vi "RT Main.vi"() -> ()   [LabVIEW 2021]
doc: "This example monitors the myRIO onboard button and increments or decrements the number below based on the Direction control."
uses:
  <vilib>/myRIO/Instrument Drivers/Utilities/Utilities.lvlib
  <vilib>/myRIO/Express VI/Onboard Devices/Button/Button Express VI.xnode
  <vilib>/myRIO/Instrument Drivers/Onboard IO/DIO/vis/Read.vi
  <vilib>/myRIO/Instrument Drivers/Onboard IO/DIO/DIO.lvlib
  <vilib>/myRIO/Common/Instrument Driver Framework/myRIO v1.0/DIO/typedefs/DIO Channels Enum.ctl
  <vilib>/myRIO/Common/Instrument Driver Framework/myRIO v1.0/DIO/typedefs/DIO Channels List.ctl
  <vilib>/myRIO/Common/Instrument Driver Framework/Utilities/typedefs/Generic FPGA Reference.ctl
  <vilib>/myRIO/Common/Instrument Driver Framework/Utilities/typedefs/myRIO v1.0 Reference.ctl
  <vilib>/myRIO/Common/Instrument Driver Framework/Utilities/typedefs/Hardware Version Enum.ctl
  <vilib>/myRIO/Common/Instrument Driver Framework/Utilities/typedefs/myRIO Generic Hardware Reference.ctl
  <vilib>/myRIO/Instrument Drivers/Onboard IO/DIO/typedefs/DIO Reference.ctl
  <vilib>/myRIO/Instrument Drivers/Onboard IO/DIO/vis/myRIO DIO Open.xnode
  <vilib>/myRIO/Common/Instrument Driver Framework/Utilities/vis/Is FPGA Ref Available.vi
  <vilib>/myRIO/Common/Instrument Driver Framework/myRIO v1.0/DIO/vis/myRIO v1.1 Open DIO.vi
  <vilib>/userdefined/High Color/nirio_resource_hc.ctl
panel:
  out "error out":errorcluster
  out "Button Value":bool
  in  "Direction":bool
  in  "Stop":bool
  out "Up/Down Counter":i32
  # "Overview: This example monitors the myRIO onboard button and increments or decrements the number below based on the Direction control.\nInstructions:\n1. Check the myRIO target IP Address in the project and make sure the target IP Address is correct.\n2. Run the VI.\n3. Push the button on the myRIO device."
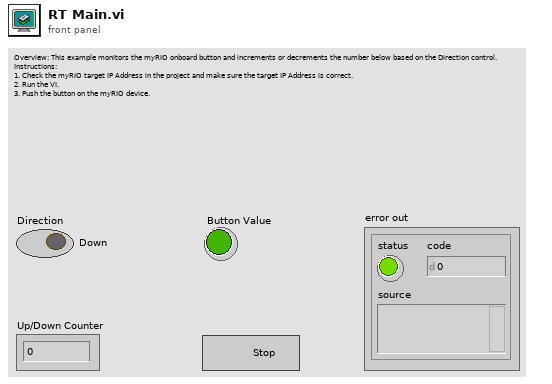
[diagram p1: front panel]
types:
  T1 = typedef "DIO.lvlib/DIO Reference.ctl" = cluster{"myRIO Reference":T2, "DIO Channels List":T6}
  T2 = typedef "myRIO Generic Hardware Reference.ctl" = cluster{"myRIO Model":T3, "myRIO Hardware Reference":T4}
  T3 = typedef "Hardware Version Enum.ctl" = enum16{"Unknown", "myRIO-1900", "myRIO-1950", "roboRIO", "NI ELVIS RIO CM", "ELVIS III"}
  T4 = typedef "myRIO v1.0 Reference.ctl" = cluster{"Generic FPGA Reference":T5, "Allow multiple opens":bool}
  T5 = typedef "Generic FPGA Reference.ctl" = refnum<k20>
  T6 = typedef "DIO Channels List.ctl" = T7[]
  T7 = typedef "DIO Channels Enum.ctl" = enum16{"Not Connected", "C/DIO0", "C/DIO1", "C/DIO2", "C/DIO3", "C/DIO4", "C/DIO5", "C/DIO6", "C/DIO7", "A/DIO0", "A/DIO1", "A/DIO2", "A/DIO3", "A/DIO4", "A/DIO5", "A/DIO6", "A/DIO7", "A/DIO8", "A/DIO9", "A/DIO10", "A/DIO11", "A/DIO12", "A/DIO13", "A/DIO14", "A/DIO15", "A/DIO16", "A/DIO17", "A/DIO18", "A/DIO19", "B/DIO0", "B/DIO1", "B/DIO2", "B/DIO3", "B/DIO4", "B/DIO5", "B/DIO6", "B/DIO7", "B/DIO8", "B/DIO9", "B/DIO10", "B/DIO11", "B/DIO12", "B/DIO13", "B/DIO14", "B/DIO15", "B/DIO16", "B/DIO17", "B/DIO18", "B/DIO19", "LED0", "LED1", "LED2", "LED3", "Button0", "DIO/DIO0", "DIO/DIO1", "DIO/DIO2", "DIO/DIO3", "DIO/DIO4", "DIO/DIO5", "DIO/DIO6", "DIO/DIO7", "DIO/DIO8", "DIO/DIO9", "SPI/CS0", "SPI/CS1", "SPI/CS2", "SPI/CS3", "LED RADIO (Green)", "LED RADIO (Red)", "LED COMM (Green)", "LED COMM (Red)", "LED MODE (Green)", "LED MODE (Red)"}
  T8 = typedef "nirio_resource_hc.ctl" = tag
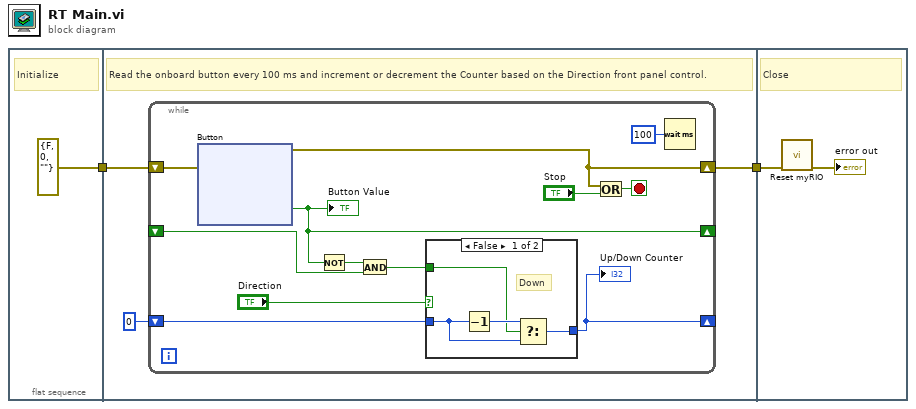
[diagram p0: block diagram]
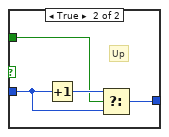
[diagram p2: hidden frame]
diagram:
  n1 = flat-sequence {
    tunnel: [errorcluster {"status"=FALSE, "code"=0, "source"=""} ("error out")] -> w1
    tunnel: [w5] -> w2
    tunnel: w1 -> [w4]
    tunnel: w2 -> [w63]
    frame #0 {
      # "Initialize"
    }
    frame #1 {
      # "Read the onboard button every 100 ms and increment or decrement the Counter based on the Direction front panel control."
      n2 = while {
        shift-right: [w12] -> _
        shift-left: 0 ("code") -> [w15]
        shift-right: [w8] -> w5
        shift-left: w4 -> [w9]
        shift-right: [w7] -> _
        shift-left: _ -> [w13]
        stop <- w18 stop-if-true
        n3 = xnode "Button"("error in (no error)"=w9) -> ("Value"=w7:bool, "error out"=w8:errorcluster)
        "Button Value" <- w7
        n4 = Not(x=w7) -> (.not. x?=w14:bool)
        n5 = And(x=w14, y=w13) -> (x .and. y?=w11:bool)
        n6 = case shown="False" "Direction" {
          tunnel: w15 -> [w56 w59]
          tunnel: [w55 w60] -> w12
          tunnel: w11 -> [w54 w58]
          frame False {
            # "Down"
            n7 = Decrement(x=w56) -> (x-1=w57:i32)
            n8 = Select(t=w57, s=w54, f=w56) -> (s? t:f=w55:i32)
          }
          frame True {
            # "Up"
            n9 = Increment(x=w59) -> (x+1=w61:i32)
            n10 = Select(t=w61, s=w58, f=w59) -> (s? t:f=w60:i32)
          }
        }
        "Up/Down Counter" <- w12
        n11 = Or(x=w8, y="Stop") -> (x .or. y?=w18:bool)
        n12 = Wait (ms)(milliseconds to wait=u32 100) -> ()  [unwired: 1 out]
      }
    }
    frame #2 {
      # "Close"
      n13 = call <vilib>:"Reset myRIO.vi"("error in (no error)"=w63) -> ("error out"=→"error out":errorcluster)  [unwired: 10 in]
    }
  }
